vi "CSB Control.vi"() -> ()   [LabVIEW 2017]
uses:
  <vilib>/Utility/error.llb/Clear Errors.vi
  <instrlib>/tio-labview/TIO Library/Data Stream/TIO Data Stream Parse Description.vi
panel:
  out "Kill":bool=TRUE
  in  "X":dbl[unit](slide)
  in  "Y":dbl[unit](slide)
  in  "Z":dbl[unit](slide)
  in  "Quit":bool
  out "ID":string="Twinleaf CSB 1.0 [7]"
  in  "URL":refnum<visa-resource-name>="tcp://localhost"
  # "CSB Control"
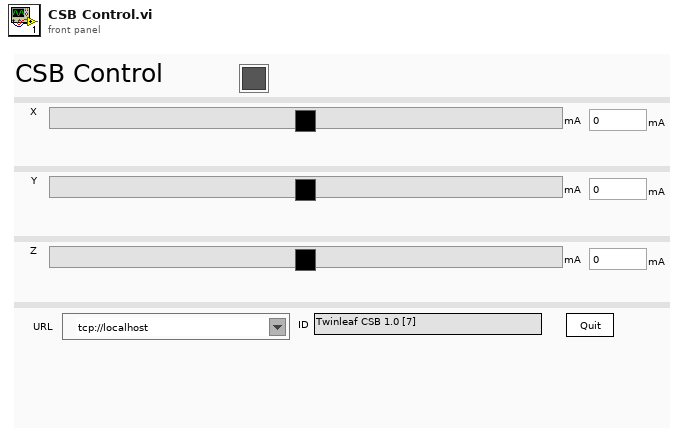
[diagram p1: front panel]
types:
  T1 = cluster{"Type":enum16{"TCP", "Serial"}, "Serial":refnum<visa-resource-name>, "TCP":refnum<k5>, "Timeout":u32}
  T2 = cluster{"Stream Description":cluster{"Stream ID":u16, "Data Type":u8, "Channels":u8, "Restart ID":u16, "Start timestamp (s)":dbl, "Sample counter":u64, "Period (s)":dbl, "Flags":u8, "Timestamp type":u8, "Name":string, "Last sample number":u64, "Last Restart ID":u16, "Version":u16, "Sample Size":u16}, "Sample #":u32, "Raw Data":string}
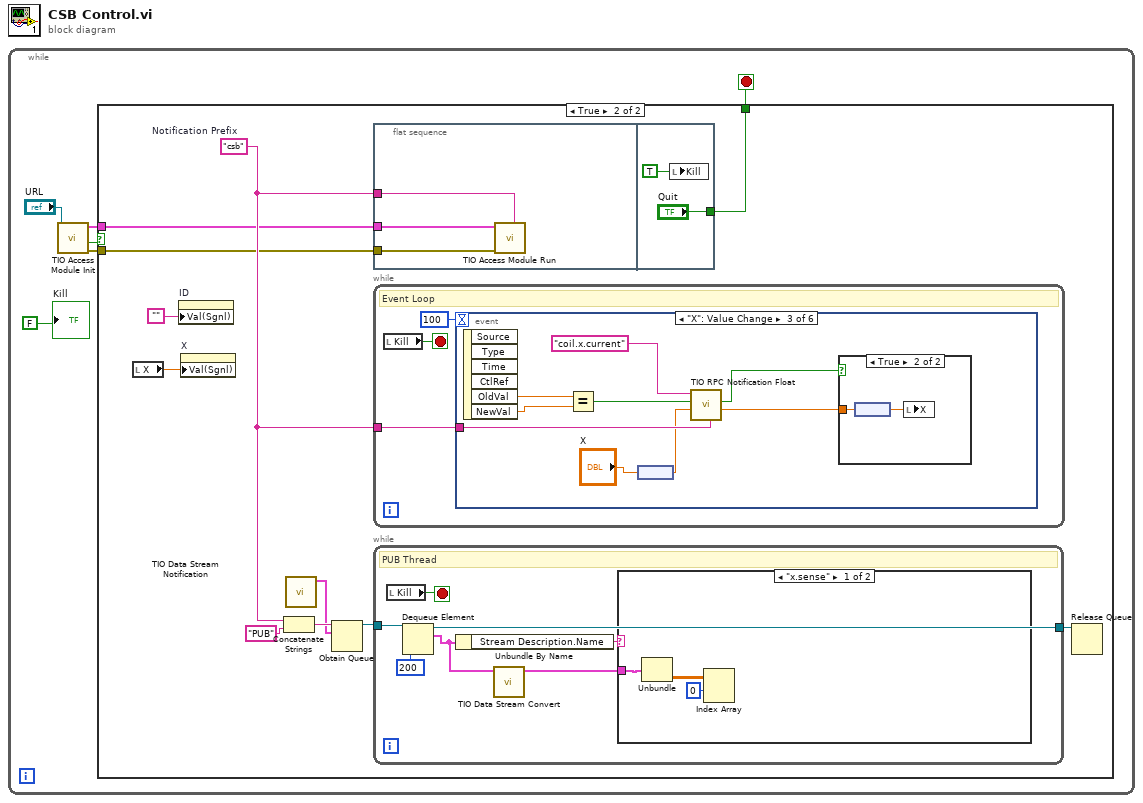
[diagram p0: block diagram]
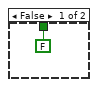
[diagram p2: hidden frame]
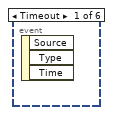
[diagram p4: hidden frame]
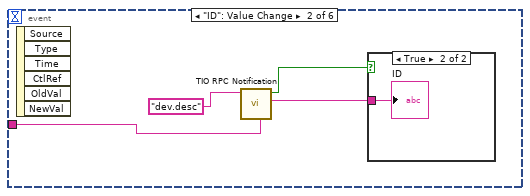
[diagram p5: hidden frame]
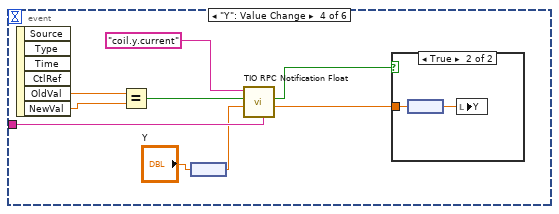
[diagram p8: hidden frame]
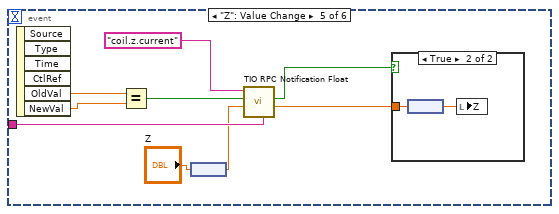
[diagram p10: hidden frame]
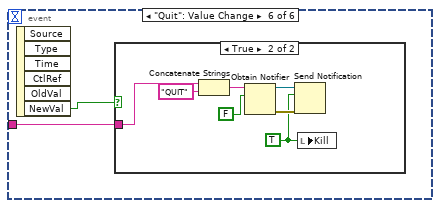
[diagram p12: hidden frame]
diagram:
  n1 = while {
    stop <- w6 stop-if-true
    n2 = call <instrlib>:"TIO Access Module Init.vi"("URL"="URL") -> ("error out"=w3:errorcluster, "Connected"=w1:bool, "TS Connection"=w4:T1)  [unwired: 8 in]
    n3 = case shown="True" w1 {
      tunnel: [FALSE ("Quit") w10] -> w6
      tunnel: w4 -> [_ w9]
      tunnel: w3 -> [_ w8]
      frame False {
      }
      frame True {
        w12 = "csb"  # Notification Prefix
        n4 = local read "X"() -> (w11:dbl[unit])
        n5 = property on="ID" class="Str"("Val(Sgnl)"="") -> ()  [unwired: 2 in, 2 out]
        n6 = property on="X" class="Slide (strict)"("Val(Sgnl)"=w11) -> ()  [unwired: 2 in, 2 out]
        n7 = Concatenate Strings(w12, "PUB" ("name (unnamed)")) -> (w17:string)
        n8 = call <instrlib>:"TIO Data Stream Notification.vi"() -> ("Data Stream Notification"=w13:T2)  [unwired: 11 in]
        n9 = Obtain Queue(name (unnamed)=w17, element data type=w13) -> (queue out=w15:refnum<queue>)  [unwired: 3 in, 2 out]
        n10 = flat-sequence {
          tunnel: w12 -> [w31]
          tunnel: w9 -> [w30]
          tunnel: w8 -> [w29]
          tunnel: ["Quit"] -> w10
          frame #0 {
            n11 = call <instrlib>:"TIO Access Module Run.vi"("Notification Prefix"=w31, "error in (no error)"=w29, "TS Connection"=w30) -> ()  [unwired: 9 in]
          }
          frame #1 {
            n12 = local write "Kill"(TRUE ("Kill")) -> ()
          }
        }
        n13 = while {
          tunnel: w12 -> [w34]
          stop <- w36 stop-if-true
          # "Event Loop"
          n14 = local read "Kill"() -> (w36:bool)
          n15 = event shown="[2] \"X\": Value Change" {
            selector: _ -> [_ _ _ _ _ _]
            dyn-events: _ -> [_ _ _ _ _ _]
            timeout: 100 -> [_ _ _ _ _ _]
            tunnel: w34 -> [_ w37 w48 w59 w70 w75]
            event Timeout {
              n16 = event-data() -> ()  [unwired: 1 in, 3 out]
            }
            event "ID": Value Change {
              n17 = event-data() -> ()  [unwired: 1 in, 6 out]
              n18 = call <instrlib>:"TIO RPC Notification.vi"("Notification Prefix"=w37, "Topic"="dev.desc") -> ("REP"=w39:string, "Response"=w38:bool)  [unwired: 6 in, 1 out]
              n19 = case shown="True" w38 {
                tunnel: w39 -> [_ w41]
                frame False {
                }
                frame True {
                  "ID" <- w41
                }
              }
            }
            event "X": Value Change {
              n20 = event-data() -> ("OldVal"=w43:dbl[unit], "NewVal"=w42:dbl[unit])  [unwired: 1 in, 4 out]
              n21 = Equal?(x=w43, y=w42) -> (x = y?=w49:bool)
              n22 = node("X") -> (w47:dbl)
              n23 = call <instrlib>:"TIO RPC Notification Float.vi"("Notification"=w48, "Set value"=w47, "Read"=w49, "String"="coil.x.current" ("Topic")) -> ("Get value (default if error)"=w46:sgl, "Response"=w45:bool)  [unwired: 4 in, 1 out]
              n24 = case shown="True" w45 {
                tunnel: w46 -> [_ w52]
                frame False {
                }
                frame True {
                  n25 = node(w52) -> (w51:sgl[unit])
                  n26 = local write "X"(w51) -> ()
                }
              }
            }
            event "Y": Value Change {
              n27 = event-data() -> ("OldVal"=w55:dbl[unit], "NewVal"=w54:dbl[unit])  [unwired: 1 in, 4 out]
              n28 = Equal?(x=w55, y=w54) -> (x = y?=w60:bool)
              n29 = node("Y") -> (w58:dbl)
              n30 = call <instrlib>:"TIO RPC Notification Float.vi"("Notification"=w59, "Set value"=w58, "Read"=w60, "String"="coil.y.current" ("Topic")) -> ("Get value (default if error)"=w57:sgl, "Response"=w56:bool)  [unwired: 4 in, 1 out]
              n31 = case shown="True" w56 {
                tunnel: w57 -> [_ w63]
                frame False {
                }
                frame True {
                  n32 = node(w63) -> (w62:sgl[unit])
                  n33 = local write "Y"(w62) -> ()
                }
              }
            }
            event "Z": Value Change {
              n34 = event-data() -> ("OldVal"=w66:dbl[unit], "NewVal"=w65:dbl[unit])  [unwired: 1 in, 4 out]
              n35 = Equal?(x=w66, y=w65) -> (x = y?=w71:bool)
              n36 = node("Z") -> (w69:dbl)
              n37 = call <instrlib>:"TIO RPC Notification Float.vi"("Notification"=w70, "Set value"=w69, "Read"=w71, "String"="coil.z.current" ("Topic")) -> ("Get value (default if error)"=w68:sgl, "Response"=w67:bool)  [unwired: 4 in, 1 out]
              n38 = case shown="True" w67 {
                tunnel: w68 -> [_ w74]
                frame False {
                }
                frame True {
                  n39 = node(w74) -> (w73:sgl[unit])
                  n40 = local write "Z"(w73) -> ()
                }
              }
            }
            event "Quit": Value Change {
              n41 = event-data() -> ("NewVal"=w76:bool)  [unwired: 1 in, 5 out]
              n42 = case shown="True" w76 {
                tunnel: w75 -> [_ w77]
                frame False {
                }
                frame True {
                  w78 = TRUE ("Kill")
                  n43 = Concatenate Strings(w77, "QUIT" ("name (unnamed)")) -> (w83:string)
                  n44 = Obtain Notifier(name (unnamed)=w83, notification data type=FALSE ("Connected")) -> (notifier out=w80:refnum<notifier>, error out=w81:errorcluster)  [unwired: 2 in, 1 out]
                  n45 = Send Notification(notification=w78, notifier=w80, error in (no error)=w81) -> ()  [unwired: 2 out]
                  n46 = local write "Kill"(w78) -> ()
                }
              }
            }
          }
        }
        n47 = while {
          tunnel: w15 -> [w24]
          tunnel: [w22] -> w14
          stop <- w25 stop-if-true
          # "PUB Thread"
          n48 = local read "Kill"() -> (w25:bool)
          n49 = Dequeue Element(queue=w24, timeout in ms (-1)=200) -> (queue out=w22:refnum<queue>, element=w19:T2)  [unwired: 1 in, 2 out]
          n50 = Unbundle By Name(w19) -> ("Stream Description.Name"=w21:string)
          n51 = call <instrlib>:"TIO Data Stream Convert.vi"("Data Stream Notification"=w19) -> ("Waveform"=w20:cluster{dbl, dbl, dbl[][]})  [unwired: 10 in]
          n52 = case shown="\"x.sense\"" w21 {
            tunnel: w20 -> [w26 _]
            frame "x.sense" {
              n53 = Unbundle(w26) -> (w27:dbl[][])  [unwired: 2 out]
              n54 = Index Array(array=w27, index (row)=0 ("disabled index (col)")) -> ()  [unwired: 1 in, 1 out]
            }
            frame Default {
            }
          }
        }
        n55 = Release Queue(queue=w14) -> ()  [unwired: 2 in, 3 out]
      }
    }
    "Kill" <- FALSE ("Kill")
  }
